vi "Degrees to left target.vi"(1 "Degrees From The Right Target":dbl, 2 "d":dbl) -> (0 "Degrees To The Left Target":dbl)   [LabVIEW 2013]
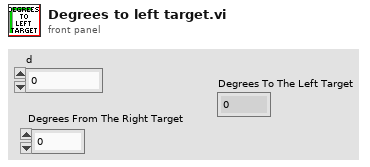
[diagram p1: front panel]
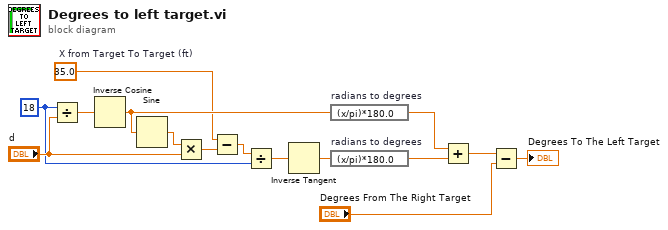
[diagram p0: block diagram]
diagram:
  w1 = 35.0  # X from Target To Target (ft)
  w10 = 18
  n1 = Divide(x=w10, y="d") -> (x/y=w15:dbl)
  n2 = Inverse Cosine(1:w15) -> (0:w7:dbl)
  n3 = Sine(x=w7) -> (sin(x)=w14:dbl)
  n4 = Multiply(x=w14, y="d") -> (x*y=w12:dbl)
  n5 = Subtract(x=w1, y=w12) -> (x-y=w11:dbl)
  n6 = Divide(x=w11, y=w10) -> (x/y=w9:dbl)
  n7 = Inverse Tangent(1:w9) -> (0:w8:dbl)
  n8 = expression code="(x/pi)*180.0" "radians to degrees"(w7) -> (w5:dbl)
  n9 = expression code="(x/pi)*180.0" "radians to degrees"(w8) -> (w6:dbl)
  n10 = Add(x=w5, y=w6) -> (x+y=w4:dbl)
  n11 = Subtract(x=w4, y="Degrees From The Right Target") -> (x-y=→"Degrees To The Left Target":dbl)
